vi "removeEmptyStrings.vi"(8 "error in (no error)":errorcluster, 11 "stringArray in":string[](array[string])) -> (0 "error out":errorcluster, 3 "stringArray out":string[](array[string]))   [LabVIEW 2018]
doc: "Remove empty strings."
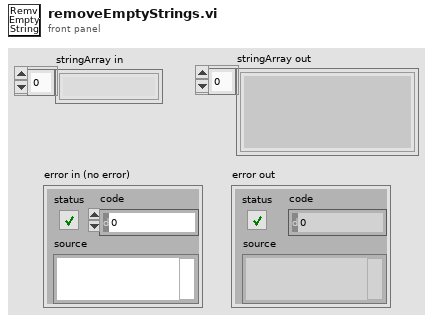
[diagram p1: front panel]
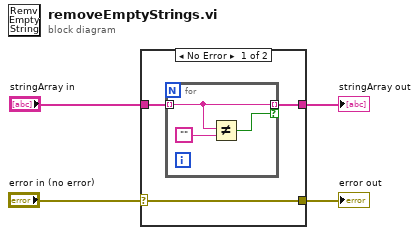
[diagram p0: block diagram]
diagram:
  n1 = case shown="No Error" "error in (no error)" {
    selector: "error in (no error)" -> [w5 w11]
    tunnel: [w7 w12] -> w4
    tunnel: "stringArray in" -> [w6 w12]
    tunnel: [w5 w11] -> w1
    frame No Error {
      n2 = for {
        tunnel: w6 -> [w9] mode=indexing
        tunnel: [w9] -> w7 mode=indexing if=w8
        n3 = Not Equal?(x=w9, y="") -> (x != y?=w8:bool)
      }
    }
    frame Error {
    }
  }
  "stringArray out" <- w4
  "error out" <- w1
